vi "HP 6643A - GPIB Monitor.vi"() -> ()   [LabVIEW 2018]
doc: "This example performs a serial port write and a serial port read. The parameters set for the serial port must match the parameters of the connected instrument or device. The VISA Configure Serial Port VI sets the configuration parameters. The front panel displays the controls used to configure the basic parameters, such as baud rate, data bits, and parity. The VI passes the VISA resource name to other VIs that perform operations on that VISA resource. The VISA Write function sends a command to the serial device and the VISA Read function returns data based on the command. The VISA Close function then closes the reference to the serial device. It is important to close the reference; otherwise, further communication through that port might not be possible."
uses:
  <vilib>/Instr/_visa.llb/VISA Open Access Mode.ctl
panel:
  out "Current (Amps)":dbl format="%.3f"
  out "Voltage (Volts)":dbl format="%.3f"
  out "Iterations":i32
  in  "stop":bool
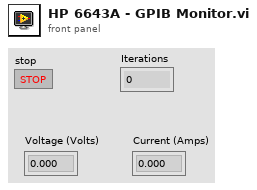
[diagram p1: front panel]
types:
  T1 = typedef "VISA Open Access Mode.ctl" = u32
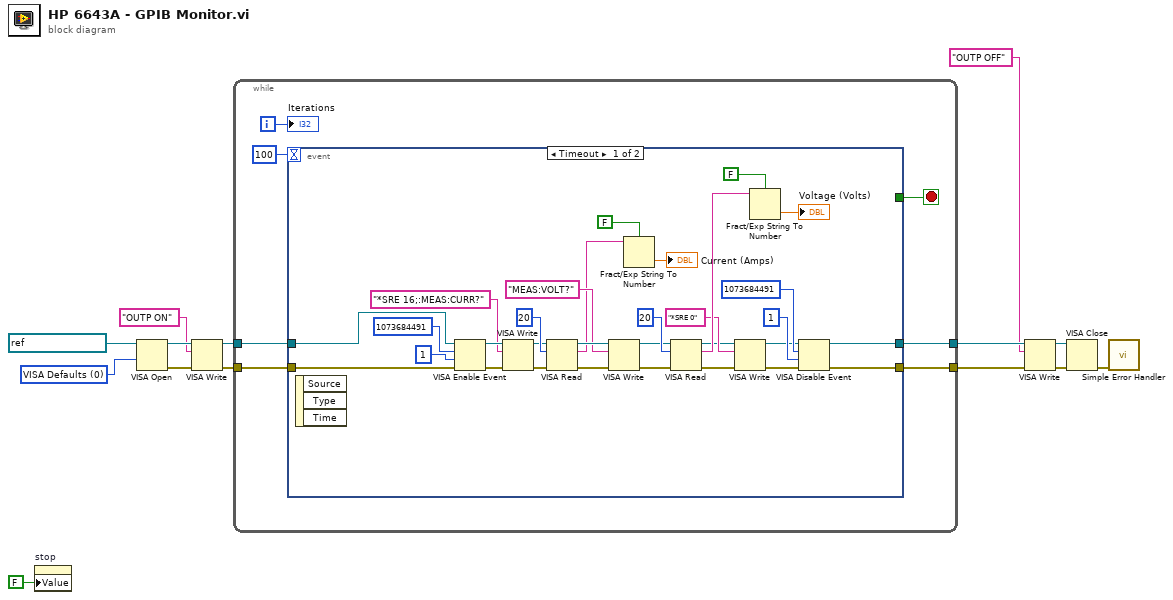
[diagram p0: block diagram]
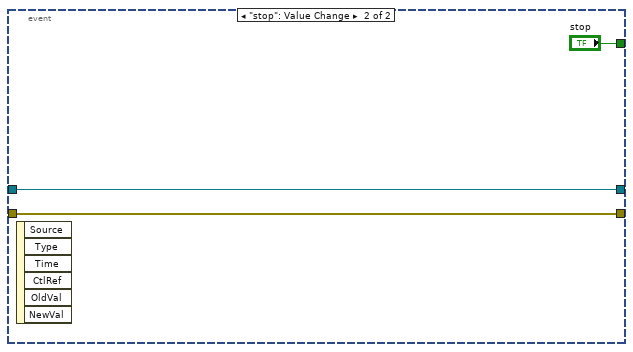
[diagram p2: hidden frame]
diagram:
  w13 = T1 0 items=["VISA Defaults"=0, "Exclusive Lock"=1, "Load Configured Settings"=4] ("Access Mode")
  n1 = property on="stop" class="Bool (strict)"("Value"=FALSE ("stop")) -> ()  [unwired: 2 in, 2 out]
  n2 = VISA Open(access mode=w13, VISA resource name=refnum<visa-resource-name> "DESK-06643A") -> (VISA resource name=w6:refnum<visa-resource-name>, error out=w7:errorcluster)  [unwired: 3 in]
  n3 = VISA Write(VISA resource name=w6, write buffer="OUTP ON", error in (no error)=w7) -> (VISA resource name out=w4:refnum<visa-resource-name>, error out=w3:errorcluster)  [unwired: 1 out]
  n4 = while {
    tunnel: w3 -> [w21]
    tunnel: w4 -> [w20]
    tunnel: [w18] -> w10
    tunnel: [w19] -> w12
    i -> [w16]
    stop <- w17 stop-if-true
    n5 = event shown="[0] Timeout" {
      selector: _ -> [_ _]
      dyn-events: _ -> [_ _]
      timeout: 100 -> [_ _]
      tunnel: w21 -> [w28 w54]
      tunnel: w20 -> [w29 w53]
      tunnel: [w26 w54] -> w19
      tunnel: [w27 w53] -> w18
      tunnel: [_ "stop"] -> w17
      event Timeout {
        n6 = event-data() -> ()  [unwired: 1 in, 3 out]
        n7 = VISA Enable Event(8:w28, 9:u16 1, 10:u32 1073684491, 11:w29) -> (0:w37:errorcluster, 3:w38:refnum<visa-resource-name>)
        n8 = VISA Write(VISA resource name=w38, write buffer="*SRE 16;:MEAS:CURR?", error in (no error)=w37) -> (VISA resource name out=w25:refnum<visa-resource-name>, error out=w24:errorcluster)  [unwired: 1 out]
        n9 = VISA Read(VISA resource name=w25, byte count=20, error in (no error)=w24) -> (VISA resource name out=w51:refnum<visa-resource-name>, read buffer=w47:string, error out=w50:errorcluster)  [unwired: 1 out]
        n10 = VISA Write(VISA resource name=w51, write buffer="MEAS:VOLT?", error in (no error)=w50) -> (VISA resource name out=w23:refnum<visa-resource-name>, error out=w22:errorcluster)  [unwired: 1 out]
        n11 = Fract/Exp String To Number(use system decimal point (T)=FALSE, string=w47) -> (number=→"Current (Amps)":dbl)  [unwired: 2 in, 1 out]
        n12 = VISA Read(VISA resource name=w23, byte count=u32 20, error in (no error)=w22) -> (VISA resource name out=w42:refnum<visa-resource-name>, read buffer=w46:string, error out=w41:errorcluster)  [unwired: 1 out]
        n13 = VISA Write(VISA resource name=w42, write buffer="*SRE 0", error in (no error)=w41) -> (VISA resource name out=w32:refnum<visa-resource-name>, error out=w33:errorcluster)  [unwired: 1 out]
        n14 = Fract/Exp String To Number(use system decimal point (T)=FALSE, string=w46) -> (number=→"Voltage (Volts)":dbl)  [unwired: 2 in, 1 out]
        n15 = VISA Disable Event(8:w33, 9:u16 1, 10:u32 1073684491, 11:w32) -> (0:w26:errorcluster, 3:w27:refnum<visa-resource-name>)
      }
      event "stop": Value Change {
        n16 = event-data() -> ()  [unwired: 1 in, 6 out]
      }
    }
    "Iterations" <- w16
  }
  n17 = VISA Write(VISA resource name=w10, write buffer="OUTP OFF", error in (no error)=w12) -> (VISA resource name out=w9:refnum<visa-resource-name>, error out=w11:errorcluster)  [unwired: 1 out]
  n18 = VISA Close(VISA resource name=w9, error in (no error)=w11) -> (error out=w14:errorcluster)
  n19 = call <vilib>:"Simple Error Handler.vi"("error in (no error)"=w14) -> ()  [unwired: 1 in, 8 out]
